vi "niRFSTS Util Option String.vi"(8 "error in (no error)":errorcluster, 11 "FPGA File Path":string="'C:\\Users\\Public\\Documents\\National Instruments\\FPGA Extensions Bitfiles\\NI PXIe-5646R\\NI-5530.lvbitx'") -> (0 "error out":errorcluster, 1 "FPGA Option String":string, 2 "FPGA Name":string, 3 "FPGA File":string)   [LabVIEW 2014]
doc: "Returns the RFSA/G Option string for a FPGA File Path."
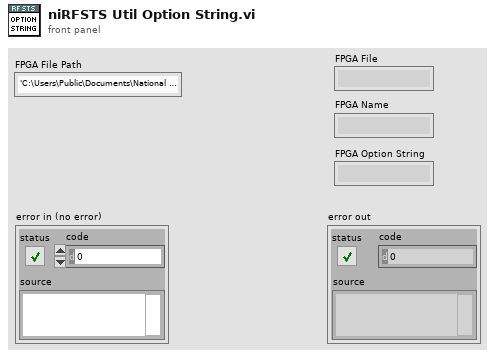
[diagram p1: front panel]
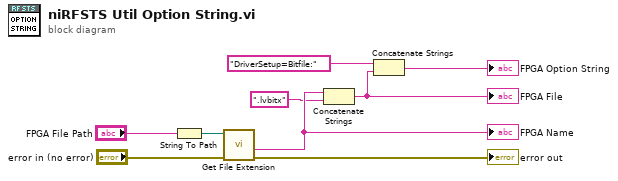
[diagram p0: block diagram]
diagram:
  n1 = String To Path(string="FPGA File Path") -> (path=w9:path)
  n2 = call <vilib>:"Get File Extension.vi"("error in (no error)"="error in (no error)", "file"=w9) -> ("error out"=→"error out":errorcluster, "filename without extension"=w6:string)  [unwired: 6 in, 2 out]
  "FPGA Name" <- w6
  n3 = Concatenate Strings(w6, ".lvbitx" ("replace string (\"\")")) -> (w3:string)
  "FPGA File" <- w3
  n4 = Concatenate Strings("DriverSetup=Bitfile:", w3) -> (→"FPGA Option String":string)
